vi "PAM.vi"(6 "PAM Control":tag="EASY9747", 9 "MASTER CONTROL":bool, 10 "?":bool, 11 "?":bool) -> ()   [LabVIEW 2017]
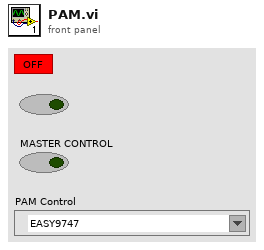
[diagram p1: front panel]
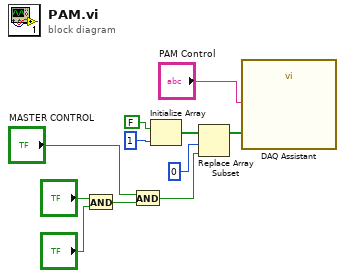
[diagram p0: block diagram]
diagram:
  n1 = And(x="?", y="?") -> (x .and. y?=w5:bool)
  n2 = And(x="MASTER CONTROL", y=w5) -> (x .and. y?=w9:bool)
  n3 = Initialize Array(FALSE, 1 ("dimension size")) -> (w7:bool[])
  n4 = Replace Array Subset(array=w7, new element=w9, index=0) -> (w10:bool[])
  n5 = call "DAQ Assistant"("data"=w10, "device name"="PAM Control") -> ()  [unwired: 16 in, 2 out]
